vi "destroy node.vi"(8 "error in":errorcluster, 11 "refnum in":T1) -> (0 "error out":errorcluster, 3 "remaining nodes alive[]":string[](array[string]))   [LabVIEW 2023, in "Publisher Subscriber.lvlib"]
uses:
  <userlib>/_Publisher Subscriber/Publisher Subscriber.lvlib
  <userlib>/_Publisher Subscriber/Controls/node refnum.ctl
  <userlib>/_Publisher Subscriber/Controls/node dvr data.ctl
  <userlib>/_Publisher Subscriber/Controls/data cluster.ctl
  <userlib>/_Publisher Subscriber/Controls/subscription bank ref.ctl
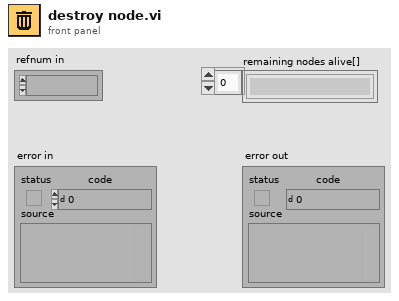
[diagram p1: front panel]
types:
  T1 = typedef "Publisher Subscriber.lvlib/node refnum.ctl" = refnum<vi>
  T2 = typedef "Publisher Subscriber.lvlib/node dvr data.ctl" = cluster{"queue ref":refnum<queue>, "Subscription Bank Ref":refnum<data-value>, "Command":string, "Data":variant, "Subscriptions []":set{string}, "Variables DVR Ref":refnum<data-value>}
  T3 = typedef "PS Design Pattern.lvlib/main dvr data.ctl" = cluster{"queue ref":refnum<queue>, "Subscription Bank Ref":refnum<data-value>, "Command":string, "Data":variant, "Subscriptions []":set{string}, "Variables DVR Ref":refnum<data-value>}
  T4 = typedef "PS Design Pattern.lvlib/subscribation bank ref.ctl" = map{string, set{refnum<queue>}}
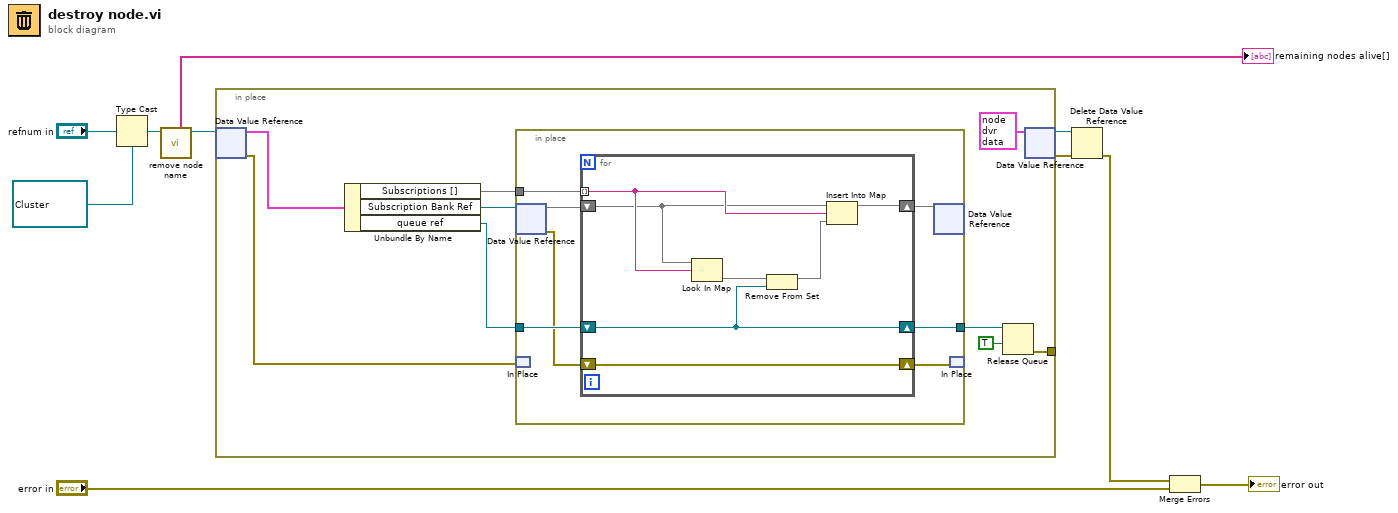
[diagram p0: block diagram]
diagram:
  n1 = Type Cast(type=refnum<data-value> refnum ("data value reference"), x="refnum in") -> (*(type *) &x=w3:refnum<data-value>)
  n2 = call <userlib>:"remove node name.vi"("Data Value Reference in"=w3) -> ("Data Value Reference out"=w2:refnum<data-value>, "nodes alive"=→"remaining nodes alive[]":string[])  [unwired: 8 in, 1 out]
  n3 = in-place {
    in-place-border: [w12] -> _
    n4 = in-place-dvr #1(w2) -> (w14:T3, w13:errorcluster)
    n5 = Unbundle By Name(w14) -> ("Subscriptions []"=w18:set{string}, "Subscription Bank Ref"=w19:refnum<data-value>, "queue ref"=w17:refnum<queue>)
    n6 = in-place {
      in-place-border: w18 -> [w24]
      in-place-border: w17 -> [w23]
      in-place-border: [w22] -> w16
      n7 = in-place-dvr #2(w19) -> (w26:T4, w20:errorcluster)
      n8 = in-place-match #3(w13) -> ()  [unwired: 1 out]
      n9 = for {
        shift-right: [w31] -> w25
        shift-left: w26 -> [w32]
        tunnel: w24 -> [w33] mode=indexing
        shift-right: [w29] -> w22
        shift-left: w23 -> [w29]
        shift-right: [w28] -> w21
        shift-left: w20 -> [w28]
        n10 = Look In Map(map=w32, key=w33) -> (value=w30:set{refnum<queue>})  [unwired: 1 in, 1 out]
        n11 = Remove From Set(10:w29, 11:w30) -> (3:w27:set{refnum<queue>})  [unwired: 1 out]
        n12 = Insert Into Map(map in=w32, key=w33, value=w27) -> (map out=w31:T4)  [unwired: 2 out]
      }
      n13 = in-place-dvr #2(w25) -> ()  [unwired: 2 out]
      n14 = in-place-match #3(w21) -> ()  [unwired: 1 out]
    }
    n15 = Release Queue(queue=w16, force destroy? (F)=TRUE) -> (error out=w12:errorcluster)  [unwired: 1 in, 2 out]
    n16 = in-place-dvr #1(T2 {"queue ref"=refnum, "Subscription Bank Ref"=refnum, "Command"="", "Data"=variant, "Subscriptions []"={}, "Variables DVR Ref"=refnum} ("data value")) -> (w8:refnum<data-value>, w5:errorcluster)
  }
  n17 = Delete Data Value Reference(data value reference=w8, error in=w5) -> (error out=w4:errorcluster)  [unwired: 1 out]
  n18 = Merge Errors(w4, "error in") -> (→"error out":errorcluster)
